vi "Size Channel Selection Arrays.vi"(8 "Error In":errorcluster, 10 "CD Settings In":T1={"CD Task Dependency"=18446744073709551615, "CD Task Dependency Ref"=18446744073709551615, "CD Task Available Wfms"=[], "CD Task Selected Wfms"=[], "Buffer Length (samples)"=0, "Number of DAQ Chanels"=0, "Min Enabled"=FALSE, "Max Enabled "=FALSE, "SP Enabled"=FALSE, "RMS Enabled"=FALSE, "Buffer Length (s)"=0.0, "Task Rate"=0.0} {"CD Task Dependency Ref" format="%.0x"; "CD Task Dependency" format="%.0x"}) -> (0 "Error Out":errorcluster, 2 "CD Settings Out":T1={"CD Task Dependency"=18446744073709551615, "CD Task Dependency Ref"=18446744073709551615, "CD Task Available Wfms"=[], "CD Task Selected Wfms"=[], "Buffer Length (samples)"=0, "Number of DAQ Chanels"=0, "Min Enabled"=FALSE, "Max Enabled "=FALSE, "SP Enabled"=FALSE, "RMS Enabled"=FALSE, "Buffer Length (s)"=0.0, "Task Rate"=0.0} {"CD Task Dependency Ref" format="%.0x"; "CD Task Dependency" format="%.0x"})   [LabVIEW 2017, in "Waveform-Processing-Custom-Device System Explorer.lvlib"]
doc: "This application will build the Arrays for the output channels.\nIF the channels have previously been defined then this process will be skipped"
uses:
  Waveform-Processing-Custom-Device System Explorer.lvlib
  <vilib>/NI Veristand/Custom Device API/Custom Device Item Ref.ctl
  <vilib>/NI VeriStand/Custom Device API/Custom Device API.lvlib
  Shared/Custom Device Settings.ctl
  Shared/Waveform-Processing-Custom-Device Shared.lvlib
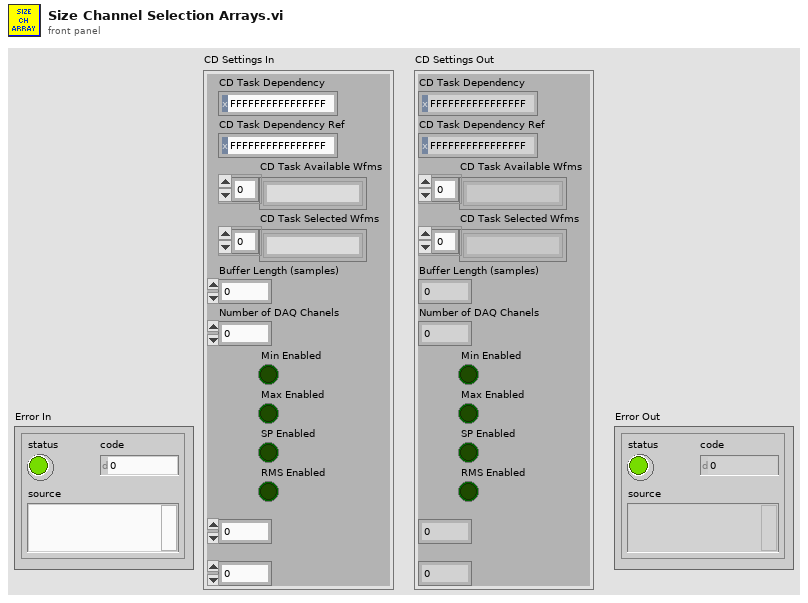
[diagram p1: front panel]
types:
  T1 = typedef "Waveform-Processing-Custom-Device Shared.lvlib/Custom Device Settings.ctl" = cluster{"CD Task Dependency":T2, "CD Task Dependency Ref":T2, "CD Task Available Wfms":string[], "CD Task Selected Wfms":string[], "Buffer Length (samples)":u32, "Number of DAQ Chanels":u32, "Min Enabled":bool, "Max Enabled ":bool, "SP Enabled":bool, "RMS Enabled":bool, "Buffer Length (s)":dbl, "Task Rate":dbl}
  T2 = typedef "Custom Device API.lvlib/Custom Device Item Ref.ctl" = u64
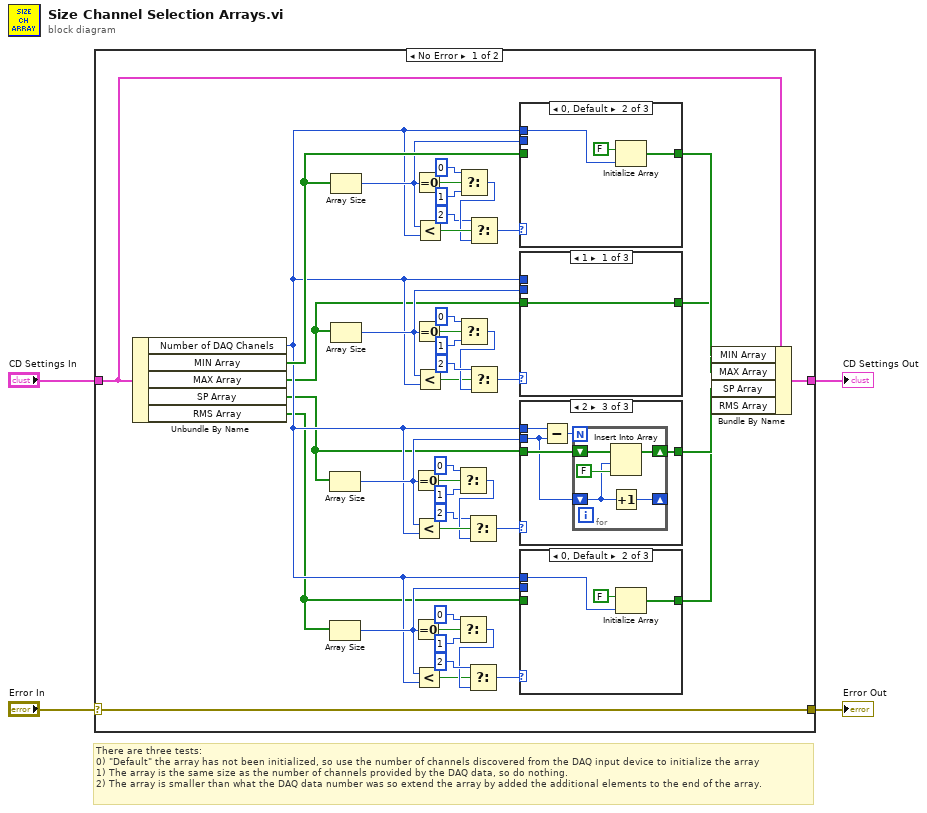
[diagram p0: block diagram]
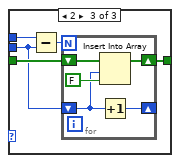
[diagram p3: hidden frame]
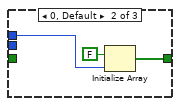
[diagram p5: hidden frame]
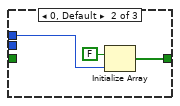
[diagram p6: hidden frame]
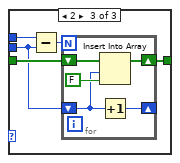
[diagram p7: hidden frame]
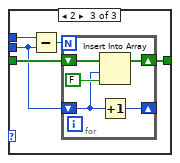
[diagram p9: hidden frame]
diagram:
  # "There are three tests:\n0)\t\"Default\" the array has not been initialized, so use the number of channels discovered from the DAQ input device to initialize the array\n1)\tThe array is the same size as the number of channels provided by the DAQ data, so do nothing.\n2)\tThe array is smaller than what the DAQ data number was so extend the array by added the additional elements to the end of the array."
  n1 = case shown="No Error" "Error In" {
    selector: "Error In" -> [w48 w106]
    tunnel: "CD Settings In" -> [w44 w105]
    tunnel: [w48 w106] -> w2
    tunnel: [w43 w105] -> w1
    frame No Error {
      n2 = Unbundle By Name(w44) -> ("Number of DAQ Chanels"=w11:u32, "MIN Array"=w42:bool[], "MAX Array"=w10:bool[], "SP Array"=w6:bool[], "RMS Array"=w5:bool[])
      n3 = Array Size(array=w6) -> (size(s)=w22:i32)
      n4 = Array Size(array=w5) -> (size(s)=w17:i32)
      n5 = Array Size(array=w42) -> (size(s)=w39:i32)
      n6 = Array Size(array=w10) -> (size(s)=w33:i32)
      n7 = Equal To 0?(x=w22) -> (x = 0?=w27:bool)
      n8 = Equal To 0?(x=w17) -> (x = 0?=w12:bool)
      n9 = Equal To 0?(x=w39) -> (x = 0?=w47:bool)
      n10 = Equal To 0?(x=w33) -> (x = 0?=w28:bool)
      n11 = Less?(x=w22, y=w11) -> (x < y?=w24:bool)
      n12 = Less?(x=w17, y=w11) -> (x < y?=w15:bool)
      n13 = Less?(x=w39, y=w11) -> (x < y?=w41:bool)
      n14 = Less?(x=w33, y=w11) -> (x < y?=w31:bool)
      n15 = Select(t=0, s=w27, f=1) -> (s? t:f=w21:i32)
      n16 = Select(t=0, s=w12, f=1) -> (s? t:f=w18:i32)
      n17 = Select(t=0, s=w47, f=1) -> (s? t:f=w37:i32)
      n18 = Select(t=0, s=w28, f=1) -> (s? t:f=w34:i32)
      n19 = Select(t=2 ("f"), s=w24, f=w21) -> (s? t:f=w23:i32)
      n20 = Select(t=2 ("f"), s=w15, f=w18) -> (s? t:f=w16:i32)
      n21 = Select(t=2 ("f"), s=w41, f=w37) -> (s? t:f=w40:i32)
      n22 = Select(t=2 ("f"), s=w31, f=w34) -> (s? t:f=w32:i32)
      n23 = case shown="0, Default" w40 {
        tunnel: w11 -> [_ w93 w96]
        tunnel: [w91 w92 w98] -> w38
        tunnel: w42 -> [w91 _ w99]
        tunnel: w39 -> [_ _ w95]
        frame 1 {
        }
        frame 0, Default {
          n24 = Initialize Array(FALSE, w93) -> (w92:bool[])
        }
        frame 2 {
          n25 = Subtract(x=w96, y=w95) -> (x-y=w97:u32)
          n26 = for {
            N: w97 -> [_]
            shift-right: [w103] -> w98
            shift-left: w99 -> [w104]
            shift-right: [w100] -> _
            shift-left: w95 -> [w101]
            n27 = Insert Into Array(array=w104, index=w101, new element=FALSE) -> (w103:bool[])
            n28 = Increment(x=w101) -> (x+1=w100:i32)
          }
        }
      }
      n29 = case shown="1" w32 {
        tunnel: w11 -> [_ w79 w82]
        tunnel: [w77 w78 w84] -> w9
        tunnel: w10 -> [w77 _ w85]
        tunnel: w33 -> [_ _ w81]
        frame 1 {
        }
        frame 0, Default {
          n30 = Initialize Array(FALSE, w79) -> (w78:bool[])
        }
        frame 2 {
          n31 = Subtract(x=w82, y=w81) -> (x-y=w83:u32)
          n32 = for {
            N: w83 -> [_]
            shift-right: [w89] -> w84
            shift-left: w85 -> [w90]
            shift-right: [w86] -> _
            shift-left: w81 -> [w87]
            n33 = Insert Into Array(array=w90, index=w87, new element=FALSE) -> (w89:bool[])
            n34 = Increment(x=w87) -> (x+1=w86:i32)
          }
        }
      }
      n35 = case shown="2" w23 {
        tunnel: w11 -> [_ w65 w68]
        tunnel: [w63 w64 w70] -> w8
        tunnel: w6 -> [w63 _ w71]
        tunnel: w22 -> [_ _ w67]
        frame 1 {
        }
        frame 0, Default {
          n36 = Initialize Array(FALSE, w65) -> (w64:bool[])
        }
        frame 2 {
          n37 = Subtract(x=w68, y=w67) -> (x-y=w69:u32)
          n38 = for {
            N: w69 -> [_]
            shift-right: [w75] -> w70
            shift-left: w71 -> [w76]
            shift-right: [w72] -> _
            shift-left: w67 -> [w73]
            n39 = Insert Into Array(array=w76, index=w73, new element=FALSE) -> (w75:bool[])
            n40 = Increment(x=w73) -> (x+1=w72:i32)
          }
        }
      }
      n41 = case shown="0, Default" w16 {
        tunnel: w11 -> [_ w51 w54]
        tunnel: [w49 w50 w56] -> w7
        tunnel: w5 -> [w49 _ w57]
        tunnel: w17 -> [_ _ w53]
        frame 1 {
        }
        frame 0, Default {
          n42 = Initialize Array(FALSE, w51) -> (w50:bool[])
        }
        frame 2 {
          n43 = Subtract(x=w54, y=w53) -> (x-y=w55:u32)
          n44 = for {
            N: w55 -> [_]
            shift-right: [w61] -> w56
            shift-left: w57 -> [w62]
            shift-right: [w58] -> _
            shift-left: w53 -> [w59]
            n45 = Insert Into Array(array=w62, index=w59, new element=FALSE) -> (w61:bool[])
            n46 = Increment(x=w59) -> (x+1=w58:i32)
          }
        }
      }
      n47 = Bundle By Name(cluster=w44, "MIN Array"=w38, "MAX Array"=w9, "SP Array"=w8, "RMS Array"=w7) -> (w43:T1)
    }
    frame Error {
    }
  }
  "Error Out" <- w2
  "CD Settings Out" <- w1
